vi "writeOutputToFile.vi"(0 "Byte Stream File in":refnum<file>, 1 "string":string, 2 "time in aqc period?":bool, 3 "save mode on?":bool) -> (5 "Byte Stream File out":refnum<file>)   [LabVIEW 2013]
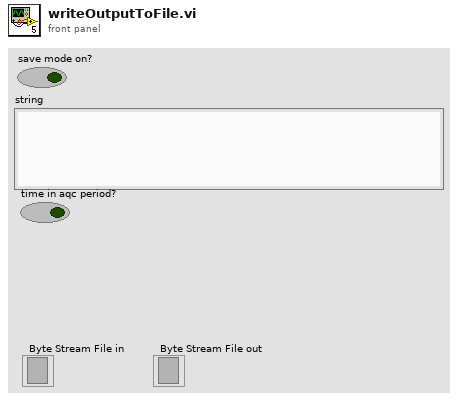
[diagram p1: front panel]
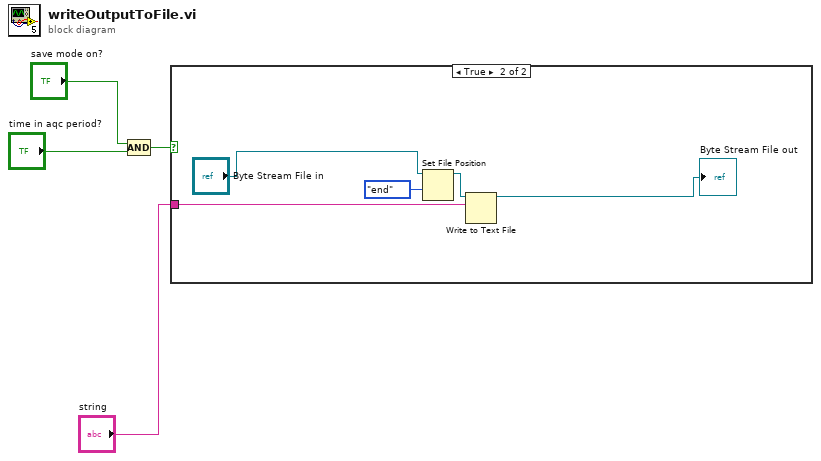
[diagram p0: block diagram]
diagram:
  n1 = Compound Arithmetic op=AND("save mode on?", "time in aqc period?") -> (w2:bool)
  n2 = case shown="True" w2 {
    tunnel: "string" -> [_ w9]
    frame False {
    }
    frame True {
      n3 = Set File Position(refnum="Byte Stream File in", from (0:start)=enum16{"start", "end", "current"}."end") -> (refnum out=w6:refnum<file>)  [unwired: 2 in, 1 out]
      n4 = Write to Text File(file (use dialog)=w6, text=w9) -> (refnum out=→"Byte Stream File out":refnum<file>)  [unwired: 2 in, 2 out]
    }
  }
